vi "Acquire & Chart RTDmap.vi"() -> ()   [LabVIEW 8.6]
uses:
  vi.lib/UeiDaq/UeiDaqCreateAISession.vi
  vi.lib/UeiDaq/UeiDaqReadOneScaledScan.vi
  <libdir>/resource/objmgr/ueidaq.rc
  vi.lib/UeiDaq/UeiDaqConfigureTimingForRTDMapIO.vi
panel:
  in  "Resources":string[](array[string])
  in  "Graph Display On":bool
  in  "Sample rate":dbl
  in  "timeout (ms)":u32
  in  "Analog Input Mode":enum16{"Differential", "Single-Ended"}(ring)
  in  "max. range (V)":dbl
  in  "min. range (V)":dbl
  out "Total scans acquired":i32
  out "Waveform Chart":dbl[][](graph)
  in  "stop":bool
  # "RTDMap analog input acquisition"
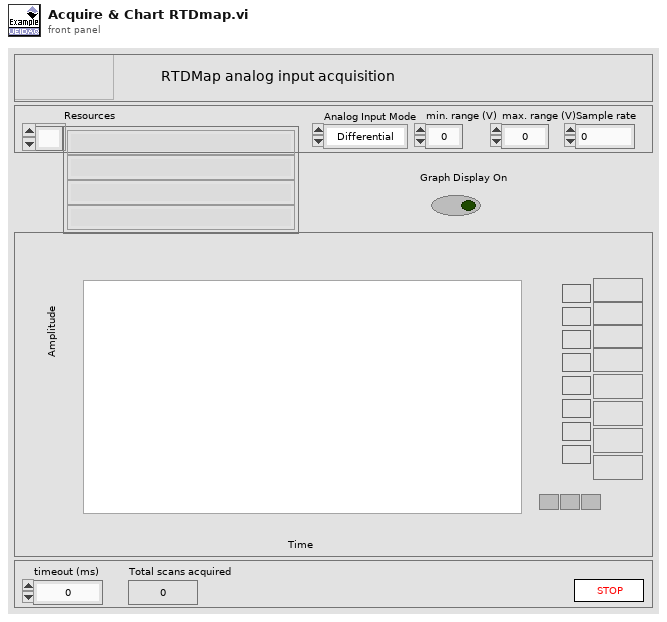
[diagram p1: front panel]
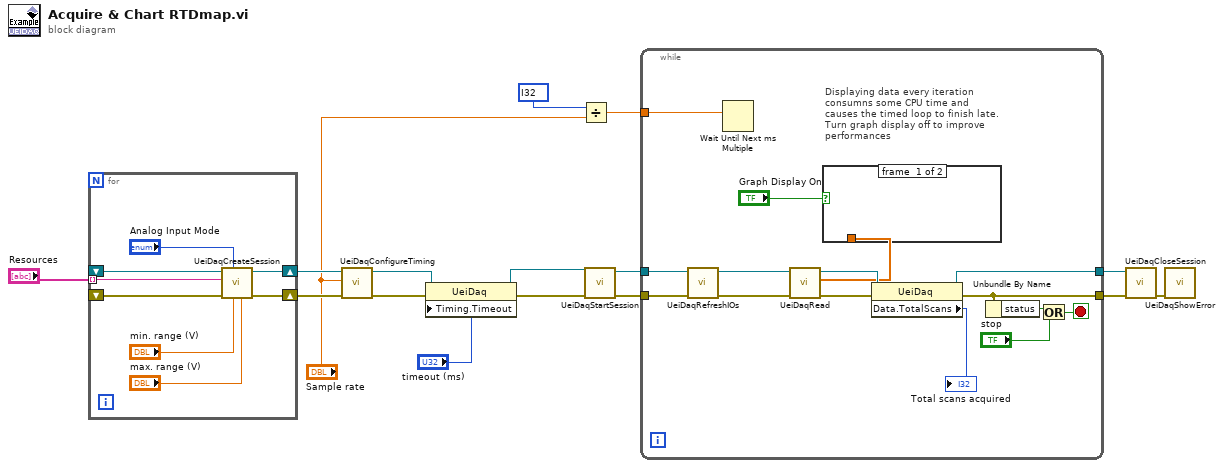
[diagram p0: block diagram]
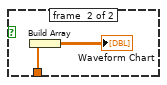
[diagram p2: hidden frame]
diagram:
  n1 = for {
    tunnel: "Resources" -> [w19] mode=indexing
    shift-right: [w23] -> w12
    shift-left: _ -> [w17]
    shift-right: [w24] -> w13
    shift-left: _ -> [w18]
    n2 = call-poly "UeiDaqCreateSession.vi"("Maximum range"="max. range (V)", "Minimum range"="min. range (V)", "Analog Input Mode"="Analog Input Mode", "error in (no error)"=w17, "Resource"=w19, "UeiDaq Refnum In"=w18) -> ("error out"=w23:errorcluster, "UeiDaq Refnum Out"=w24:refnum<k20>)  [unwired: 4 in]
  }
  n3 = call-poly "UeiDaqConfigureTiming.vi"("error in (no error)"=w12, "Rate"="Sample rate", "UeiDaq Refnum In"=w13) -> ("error out"=w11:errorcluster, "UeiDaq Refnum Out"=w10:refnum<k20>)  [unwired: 7 in]
  n4 = property class="UeiDaq"(reference=w10, error in=w11, "Timing.Timeout"="timeout (ms)") -> (reference out=w6:refnum<k20>, error out=w8:errorcluster)
  n5 = Divide(x=i32 ?, y="Sample rate") -> (x/y=w1:dbl)
  n6 = call "UeiDaqStartSession.vi"("error in (no error)"=w8, "UeiDaq Refnum In"=w6) -> ("error out"=w7:errorcluster, "UeiDaq Refnum Out"=w5:refnum<k20>)  [unwired: 8 in]
  n7 = while {
    tunnel: w5 -> [w28]
    tunnel: w7 -> [w27]
    tunnel: [w34] -> w14
    tunnel: [w33] -> w15
    tunnel: w1 -> [w29]
    stop <- w37 stop-if-true
    # "Displaying data every iteration\nconsumns some CPU time and\ncauses the timed loop to finish late.\nTurn graph display off to improve\nperformances"
    n8 = call "UeiDaqRefreshIOs.vi"("error in (no error)"=w27, "UeiDaq Refnum In"=w28) -> ("error out"=w25:errorcluster, "UeiDaq Refnum Out"=w26:refnum<k20>)  [unwired: 8 in]
    n9 = Wait Until Next ms Multiple(millisecond multiple=w29) -> ()  [unwired: 1 out]
    n10 = call-poly "UeiDaqRead.vi"("error in (no error)"=w25, "UeiDaq Refnum In"=w26) -> ("error out"=w35:errorcluster, "Scaled Data"=w31:dbl[], "UeiDaq Refnum Out"=w36:refnum<k20>)  [unwired: 7 in]
    n11 = case shown="True" "Graph Display On" {
      tunnel: w31 -> [_ w41]
      frame #0 {
      }
      frame #1 {
        n12 = Build Array(w41) -> (→"Waveform Chart":dbl[][])
      }
    }
    n13 = property class="UeiDaq"(reference=w36, error in=w35) -> (reference out=w33:refnum<k20>, error out=w34:errorcluster, "Data.TotalScans"=→"Total scans acquired":u32)
    n14 = Unbundle By Name(w34) -> ("status"=w39:bool)
    n15 = Or(x=w39, y="stop") -> (x .or. y?=w37:bool)
  }
  n16 = call "UeiDaqCloseSession.vi"("error in (no error)"=w14, "UeiDaq Refnum In"=w15) -> ("error out"=w16:errorcluster)  [unwired: 8 in, 1 out]
  n17 = call "UeiDaqShowError.vi"("error in (no error)"=w16) -> ()  [unwired: 10 in, 1 out]
